vi "ReadObjectLayout.vi"(7 "properties to ignore":variant, 8 "error in (no error)":errorcluster, 10 "GObj Refnum":refnum<vi>, 11 "NumericWithScale Control Layout in":refnum<class "NumericWithScale Control Layout.lvclass">) -> (0 "error out":errorcluster, 3 "NumericWithScale Control Layout out":refnum<class "NumericWithScale Control Layout.lvclass">)   [LabVIEW 2010, in "NI_SE_Front Panel Layout.lvlib" / "NumericWithScale Control Layout.lvclass"]
doc: "Read layout information from the GObj Refnum."
uses:
  NumericWithScale Control Layout.lvclass
  Control Layout/Control Layout.lvclass
  Digital Control Layout/Digital Control Layout.lvclass
  NumericWithScale Control Layout.lvclass/NumericWithScale Control Layout.ctl
  NI_SE_Front Panel Layout.lvlib
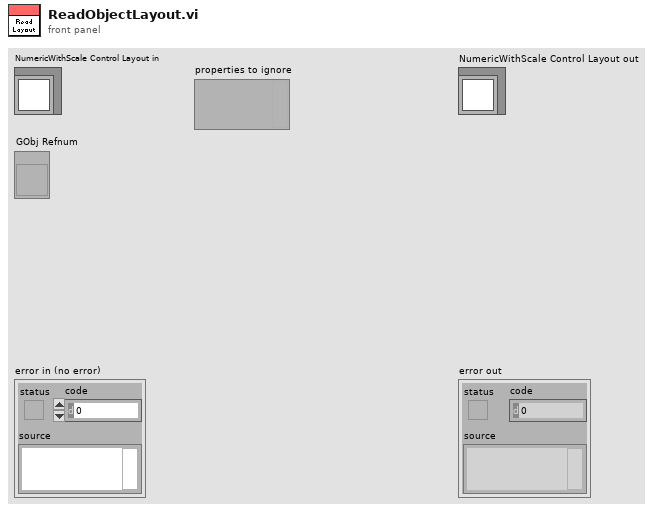
[diagram p1: front panel]
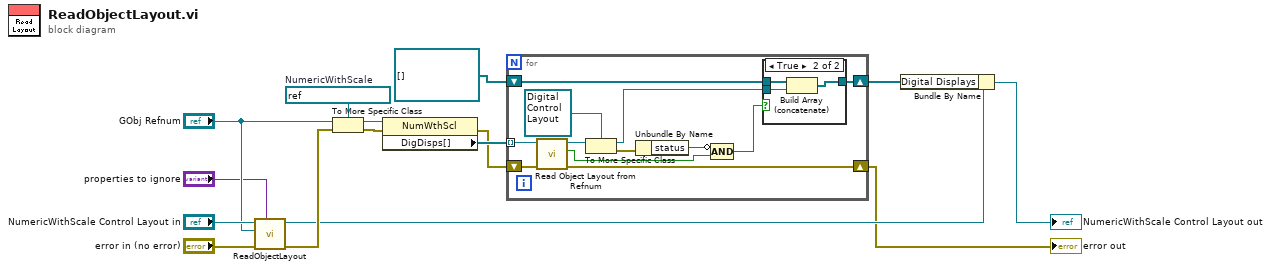
[diagram p0: block diagram]
diagram:
  w7 = refnum<vi> refnum  # NumericWithScale
  n1 = call-parent "ReadObjectLayout.vi"("properties to ignore"="properties to ignore", "error in (no error)"="error in (no error)", "GObj Refnum"="GObj Refnum", "Control Layout in"="NumericWithScale Control Layout in") -> ("error out"=w13:errorcluster, "Control Layout out"=w12:refnum<class "NumericWithScale Control Layout.lvclass">)  [unwired: 6 in]
  n2 = To More Specific Class(target class=w7, reference="GObj Refnum", error in=w13) -> (specific class reference=w6:refnum<vi>, error out=w5:errorcluster)
  n3 = property class="NumWthScl"(reference=w6, error in=w5) -> (error out=w3:errorcluster, "DigDisps[]"=w4:refnum<vi>[])  [unwired: 1 out]
  n4 = for {
    tunnel: w4 -> [w27] mode=indexing
    shift-right: [w26] -> w9
    shift-left: w3 -> [w25]
    shift-right: [w17] -> w2
    shift-left: refnum<class "Digital Control Layout.lvclass">[] [] ("Array") -> [w18]
    n5 = call "Read Object Layout from Refnum.vi"("error in"=w25, "GObj refnum"=w27) -> ("error out"=w26:errorcluster, "found?"=w21:bool, "object layout"=w23:refnum<class "Object Layout.lvclass">)  [unwired: 7 in]
    n6 = To More Specific Class(target class=refnum<class "Digital Control Layout.lvclass"> refnum ("NI_SE_Front Panel Layout.lvlib:Digital Control Layout.lvclass"), reference=w23) -> (specific class reference=w22:refnum<class "Digital Control Layout.lvclass">, error out=w19:errorcluster)  [unwired: 1 in]
    n7 = Unbundle By Name(w19) -> ("status"=w16:bool)
    n8 = Compound Arithmetic op=AND(invert w16, w21) -> (w20:bool)
    n9 = case shown="True" w20 {
      tunnel: w18 -> [w28 w30]
      tunnel: w22 -> [_ w29]
      tunnel: [w28 w31] -> w17
      frame False {
      }
      frame True {
        n10 = Build Array (concatenate)(w30, w29) -> (w31:refnum<class "Digital Control Layout.lvclass">[])
      }
    }
  }
  "error out" <- w9
  n11 = Bundle By Name(cluster=w12, "Digital Displays"=w2) -> (→"NumericWithScale Control Layout out":refnum<class "NumericWithScale Control Layout.lvclass">)
